vi "GlobalConnectTF.vi"() -> ()   [LabVIEW 2020]
panel:
  in  "Connected TF":bool
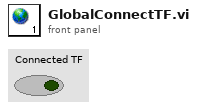
[diagram p1: front panel]
diagram:
